vi "ADC_main.vi"() -> ()   [LabVIEW 2013]
uses:
  <vilib>/Platform/TimedLoop/XDataNode/timing_clust.ctl
  <vilib>/Platform/TimedLoop/XDataNode/nitl_modes.ctl
  <vilib>/Platform/TimedLoop/XDataNode/wakeup.ctl
  <vilib>/rvi/Emulation/niFpgaSctlEmulationGetInTimedLoop.vi
  <vilib>/rvi/Emulation/niFpgaEmulationReportErrorSimple.vi
  <vilib>/rvi/Emulation/niFpgaGetClockAttributes.vi
  <vilib>/rvi/Emulation/niFpgaCriticalErrorInLSC.vi
  <vilib>/rvi/FIFO/Fifo_Resource/nirvififoEmulationWriteFpgaImpl.vi
  <vilib>/rvi/DataTransferAndStorage/Container/Common/niFpgaContainerGetUniqueNameForEmu.vi
  <vilib>/rvi/FIFO/Fifo_Resource/nirvififoEmulationReadFpgaImpl.vi
  <vilib>/rvi/Emulation/niFpgaProcessEmulError.vi
  <vilib>/rvi/FIFO/Fifo_Resource/nirvififoEmulationClearFpgaImpl.vi
  <vilib>/rvi/FIFO/Fifo_Resource/nirvififoEmulationGetNumberOfElementsToReadFpgaImpl.vi
  <vilib>/Platform/TimedLoop/XDataNode/XDataNode.xnode
  <vilib>/rvi/DataTransferAndStorage/Container/XNode/niFpgaContainer.xnode
  <vilib>/rvi/FIFO/Fifo_Resource/nirvififoEmulationWrite.vi
  <vilib>/rvi/FIFO/Fifo_Resource/nirvififoEmulationRead.vi
  <vilib>/rvi/FIFO/Fifo_Resource/nirvififoEmulationClear.vi
  <vilib>/rvi/FIFO/Fifo_Resource/nirvififoEmulationGetNumberOfElementsToRead.vi
  <vilib>/Platform/TimedLoop/XDataNode/XDNodeRunTimeDep.lvlib
panel:
  out "Timed out":bool
  out "Config":u16[](array[numeric])
  out "temp FIFO":u32
  out "config FIFO":u32
  out "output":bool
  out "ticks":i32
  out "acqu loops 2":i16
  out "avg loop":i16
  out "acqu loops":i16
  out "Number of Elements to Read":u32
  out "Data [i]":fxp<+/-,26,5>
  in  "trigger resets":i32
  in  "clock resets":i32
  in  "manual trigger":bool
  in  "acquisition":bool
  in  "get order":bool
  in  "order in":u64=434597364041252864
  in  "mode":enum16{"ramp", "RT"}(ring)=enum."RT"
  in  "avg on":bool
  out "err 2":errorcluster
  in  "Nchannels":u32=2
  out "err 1":errorcluster
  in  "avg per pt":u32=10
  out "trigged":bool
  in  "edge":enum8{"falling", "rising", "both"}(ring)=enum."both"
  in  "Trigger":i16
  in  "samples to read":u32=6
  in  "stop":bool=TRUE
  in  "clock divider":u32=160
  out "clock tick":bool
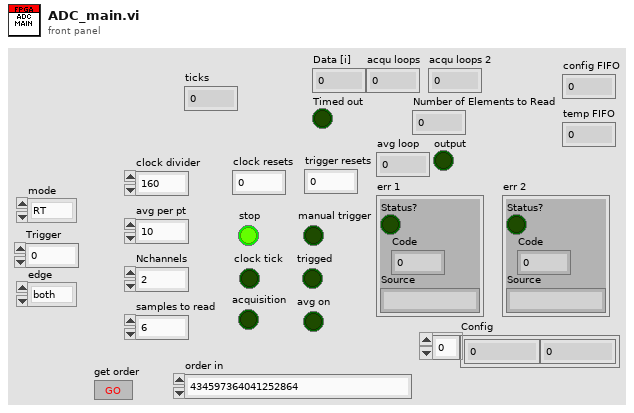
[diagram p1: front panel]
types:
  T1 = typedef "XDNodeRunTimeDep.lvlib/timing_clust.ctl" = cluster{"Expected End [f-1]":u64, "Actual End [f-1]":u64, "Finished Late? [f-1]":bool, "Expected End [i-1]":u64, "Actual End [i-1]":u64, "Finished Late? [i-1]":bool, "Expected Start [i]":u64, "Actual Start [i]":u64, "Expected Start [f]":u64, "Actual Start [f]":u64, "Source Name":string, "Structure Name":string, "Period":i64, "Deadline":i64, "Offset":i64, "Start":i64, "Priority":i32, "Timeout":i32, "Mode":T2, "Wakeup Reason":T3, "Error":errorcluster, "Source Type":string, "Secondary Source Type":string, "Global End Time":u64, "Global Start Time":u64, "Frame Duration":u64, "Iteration Duration":u64, "Assigned CPU":i32, "I/O Scan Engine Mode":u32}
  T2 = typedef "XDNodeRunTimeDep.lvlib/nitl_modes.ctl" = enum32{"No Change", "Process missed periods, maintain original phase", "Discard missed periods, maintain original phase", "Process missed periods, ignore original phase", "Discard missed periods, ignore original phase"}
  T3 = typedef "XDNodeRunTimeDep.lvlib/wakeup.ctl" = enum32{"Normal", "Aborted", "Asynchronous wakeup", "Timing source error", "Timed loop error", "Timeout"}
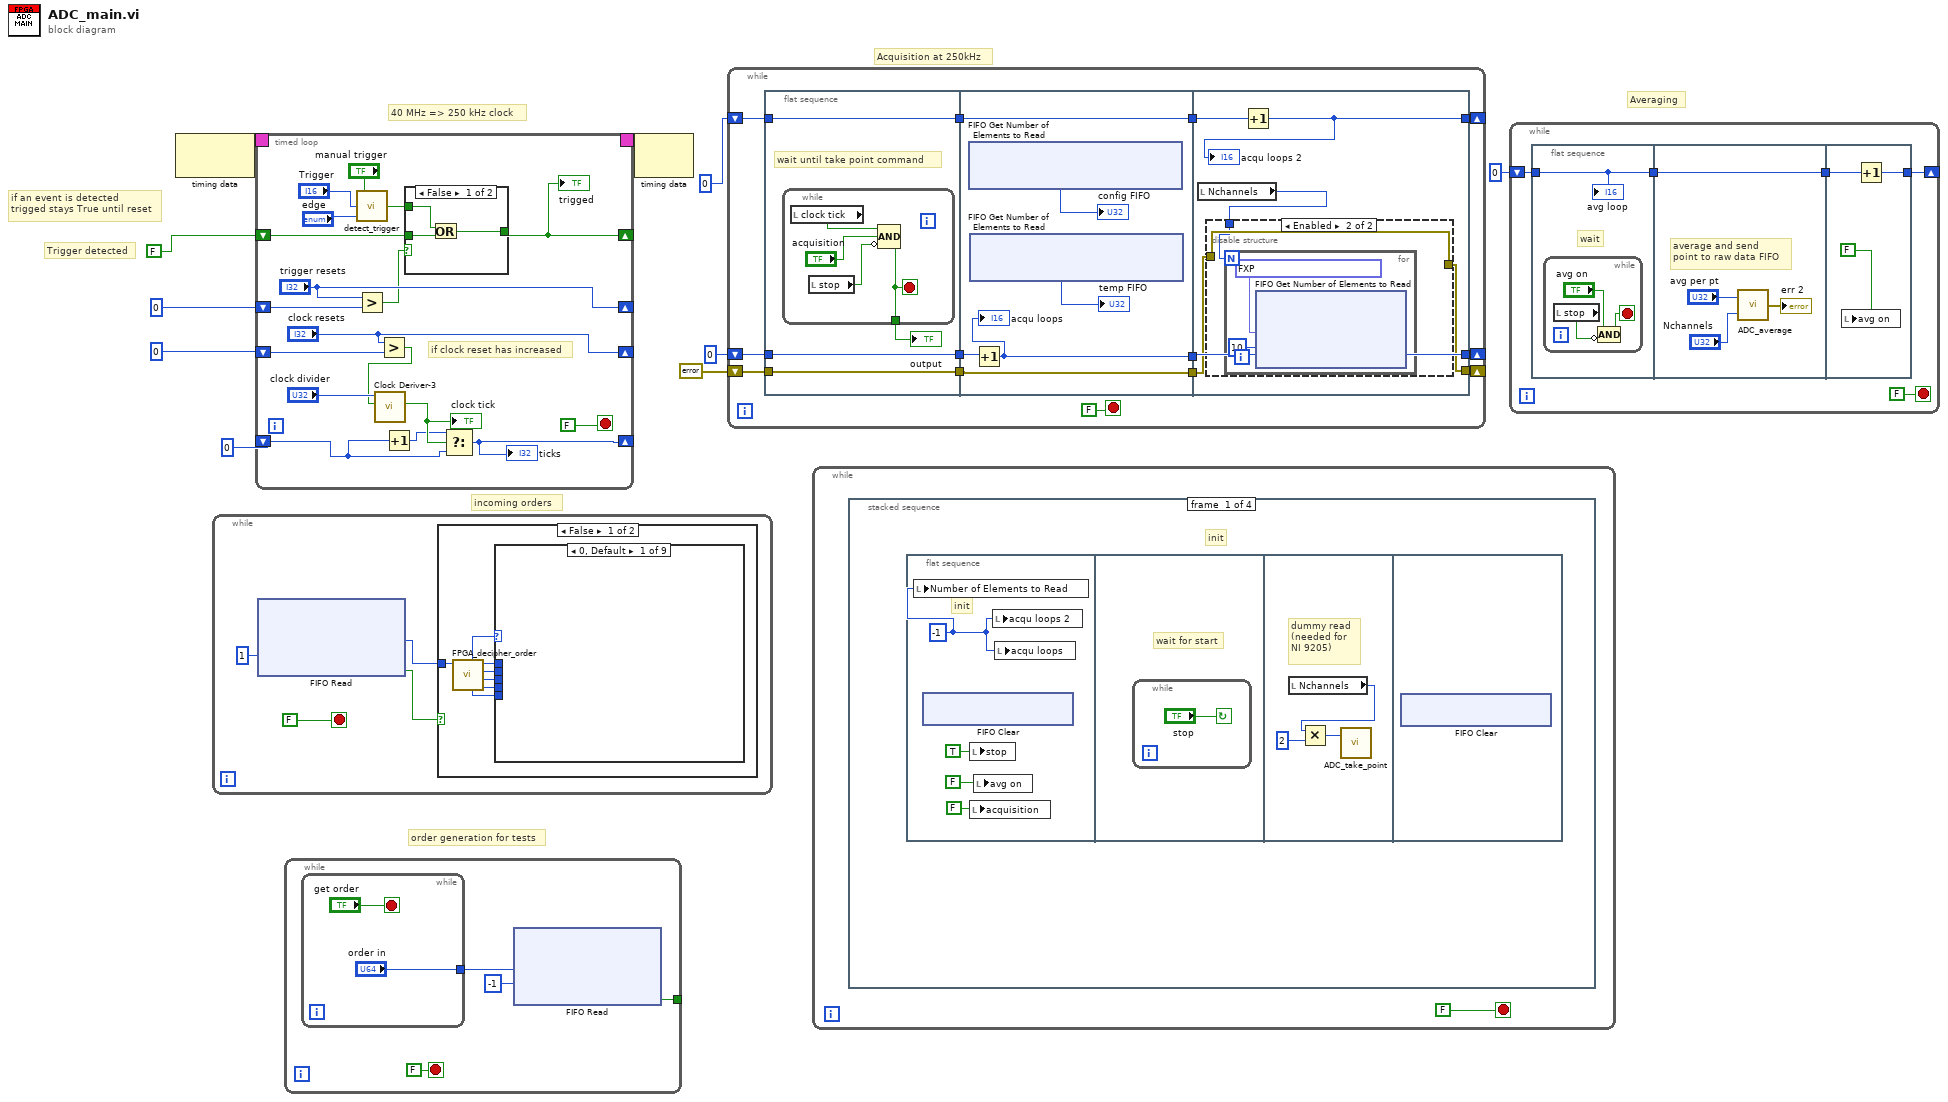
[diagram p0: block diagram]
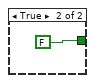
[diagram p2: hidden frame]
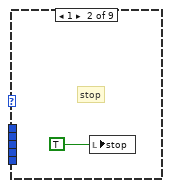
[diagram p3: hidden frame]
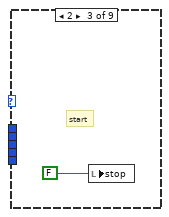
[diagram p4: hidden frame]
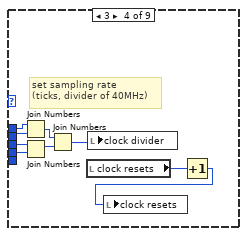
[diagram p5: hidden frame]
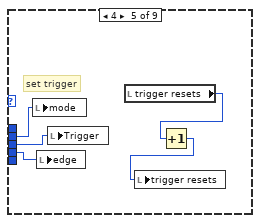
[diagram p6: hidden frame]
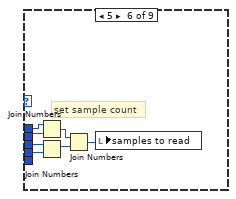
[diagram p7: hidden frame]
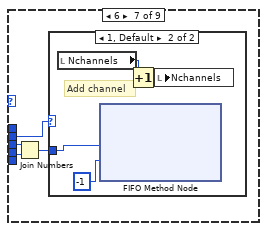
[diagram p8: hidden frame]
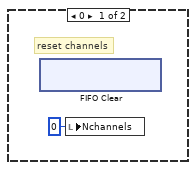
[diagram p9: hidden frame]
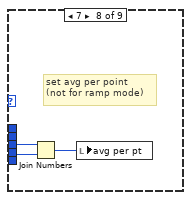
[diagram p10: hidden frame]
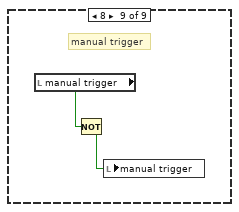
[diagram p11: hidden frame]
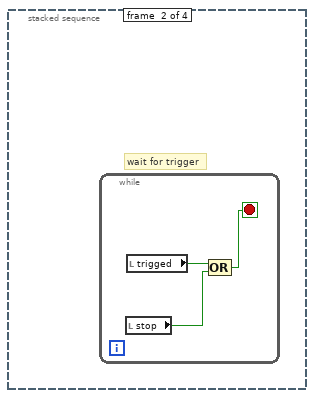
[diagram p13: hidden frame]
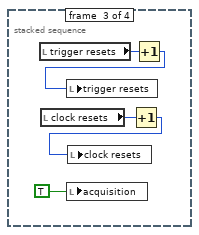
[diagram p14: hidden frame]
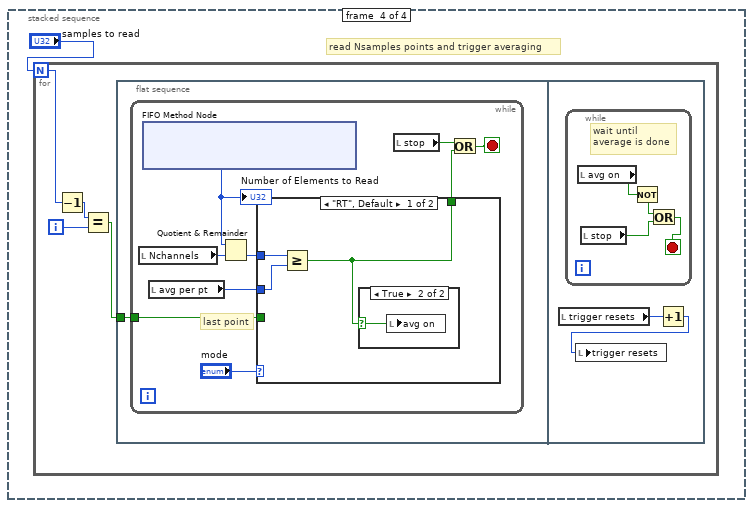
[diagram p15: hidden frame]
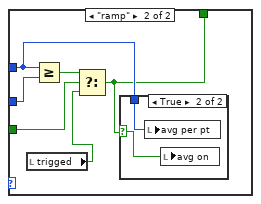
[diagram p17: hidden frame]
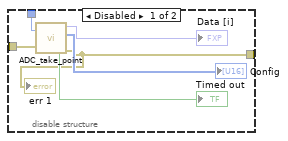
[diagram p19: hidden frame]
diagram:
  # "if an event is detected\ntrigged stays True until reset"
  # "Trigger detected"
  # "40 MHz => 250 kHz clock"
  # "incoming orders"
  # "order generation for tests"
  # "Averaging"
  # "Acquisition at 250kHz"
  n1 = node-c288() -> (w10:T1)  [unwired: 1 in]
  n2 = while {
    stop <- FALSE stop-if-true
    n3 = xnode ("FIFO Read")("Timeout"=1) -> ("Element"=w13:u64, "Timed Out?"=w11:bool)  [unwired: 1 in, 1 out]
    n4 = case shown="False" w11 {
      tunnel: w13 -> [w15 _]
      frame False {
        n5 = call "FPGA_decipher_order.vi"("order in"=w15) -> ("data 1"=w20:u8, "data 2"=w19:u8, "data 3"=w17:u8, "data 4"=w18:u8, "RFU 2"=w16:u8, "order out"=w21:u8)  [unwired: 5 out]
        n6 = case shown="0, Default" w21 {
          tunnel: w20 -> [_ _ _ w31 w37 w43 w47 w55 _]
          tunnel: w19 -> [_ _ _ w32 w35 w44 w48 w56 _]
          tunnel: w18 -> [_ _ _ w30 _ w42 _ _ _]
          tunnel: w17 -> [_ _ _ w29 w36 w41 w45 _ _]
          tunnel: w16 -> [_ _ _ _ _ _ _ _ _]
          frame 0, Default {
          }
          frame 1 {
            # "stop"
            n7 = local write "stop"(TRUE ("Stop seq")) -> ()
          }
          frame 2 {
            # "start"
            n8 = local write "stop"(FALSE ("Stop seq")) -> ()
          }
          frame 3 {
            # "set sampling rate \n(ticks, divider of 40MHz)"
            n9 = Join Numbers(hi=w30, lo=w29) -> ((hi.lo)=w28:u16)
            n10 = Join Numbers(hi=w32, lo=w31) -> ((hi.lo)=w27:u16)
            n11 = Join Numbers(hi=w28, lo=w27) -> ((hi.lo)=w26:u32)
            n12 = local read "clock resets"() -> (w25:i32)
            n13 = local write "clock divider"(w26) -> ()
            n14 = Increment(x=w25) -> (x+1=w24:i32)
            n15 = local write "clock resets"(w24) -> ()
          }
          frame 4 {
            # "set trigger"
            n16 = local write "mode"(w36) -> ()
            n17 = local write "edge"(w37) -> ()
            n18 = local write "Trigger"(w35) -> ()
            n19 = local read "trigger resets"() -> (w34:i32)
            n20 = Increment(x=w34) -> (x+1=w33:i32)
            n21 = local write "trigger resets"(w33) -> ()
          }
          frame 5 {
            # "set sample count"
            n22 = Join Numbers(hi=w42, lo=w41) -> ((hi.lo)=w40:u16)
            n23 = Join Numbers(hi=w44, lo=w43) -> ((hi.lo)=w39:u16)
            n24 = Join Numbers(hi=w40, lo=w39) -> ((hi.lo)=w38:u32)
            n25 = local write "samples to read"(w38) -> ()
          }
          frame 6 {
            n26 = Join Numbers(hi=w48, lo=w47) -> ((hi.lo)=w46:u16)
            n27 = case shown="1, Default" w45 {
              tunnel: w46 -> [_ w52]
              frame 0 {
                # "reset channels"
                n28 = xnode ("FIFO Clear")() -> ()  [unwired: 1 in, 1 out]
                n29 = local write "Nchannels"(0 ("Nchannels")) -> ()
              }
              frame 1, Default {
                # "Add channel"
                n30 = local read "Nchannels"() -> (w50:u32)
                n31 = xnode ("FIFO Method Node")("Element"=w52, "Timeout"=-1) -> ()  [unwired: 2 in, 3 out]
                n32 = Increment(x=w50) -> (x+1=w51:u32)
                n33 = local write "Nchannels"(w51) -> ()
              }
            }
          }
          frame 7 {
            # "set avg per point\n(not for ramp mode)"
            n34 = Join Numbers(hi=w56, lo=w55) -> ((hi.lo)=w54:u16)
            n35 = local write "avg per pt"(w54) -> ()
          }
          frame 8 {
            # "manual trigger"
            n36 = local read "manual trigger"() -> (w58:bool)
            n37 = Not(x=w58) -> (.not. x?=w57:bool)
            n38 = local write "manual trigger"(w57) -> ()
          }
        }
      }
      frame True {
      }
    }
  }
  n39 = timed-loop {
    timing: w10 -> [_]
    timing-out: [_] -> w9
    shift-right: [w74] -> _
    shift-left: FALSE ("reset trigger") -> [w75]
    shift-right: ["clock resets"] -> _
    shift-left: 0 ("clock resets") -> [w68]
    shift-right: ["trigger resets"] -> _
    shift-left: 0 ("trigger resets") -> [w65]
    shift-right: [w59] -> _
    shift-left: 0 -> [w60]
    stop <- FALSE stop-if-true
    # "if clock reset has increased"
    n40 = call "detect_trigger.vi"("edge"="edge", "trigger"="Trigger", "manual trigger"="manual trigger") -> ("trigged"=w73:bool)
    n41 = Greater?(x="trigger resets", y=w65) -> (0:w63:bool)
    n42 = Greater?(x="clock resets", y=w68) -> (0:w67:bool)
    n43 = call "Clock Deriver-3.vi"("reset"=w67, "Divisor"="clock divider") -> ("Clock Out"=w62:bool)  [unwired: 9 in]
    "clock tick" <- w62
    n44 = Increment(x=w60) -> (x+1=w61:i32)
    n45 = case shown="False" w63 {
      tunnel: w73 -> [w79 _]
      tunnel: w75 -> [w78 _]
      tunnel: [w77 FALSE] -> w74
      frame False {
        n46 = Or(x=w79, y=w78) -> (x .or. y?=w77:bool)
      }
      frame True {
      }
    }
    "trigged" <- w74
    n47 = Select(t=w61, s=w62, f=w60) -> (s? t:f=w59:i32)
    "ticks" <- w59
  }
  n48 = while {
    tunnel: [w83] -> _
    stop <- FALSE stop-if-true
    n49 = while {
      tunnel: ["order in"] -> w84
      stop <- "get order" stop-if-true
    }
    n50 = xnode ("FIFO Read")("Element"=w84, "Timeout"=-1) -> ("Timed Out?"=w83:bool)  [unwired: 1 in, 1 out]
  }
  n51 = node-c288(w9) -> ()  [unwired: 1 out]
  n52 = while {
    shift-right: [w99] -> _
    shift-left: i16 0 -> [w100]
    shift-right: [w93] -> _
    shift-left: i16 0 -> [w98]
    shift-right: [w92] -> _
    shift-left: errorcluster {"Status?"=FALSE, "Code"=0, "Source"=""} ("err out") -> [w90]
    stop <- FALSE stop-if-true
    n53 = flat-sequence {
      tunnel: [w105] -> w97
      tunnel: w100 -> [w105]
      tunnel: w98 -> [w103]
      tunnel: [w103] -> w95
      tunnel: w90 -> [w102]
      tunnel: [w102] -> w89
      tunnel: w97 -> [w115]
      tunnel: [w115] -> w96
      tunnel: w95 -> [w114]
      tunnel: [w113] -> w94
      tunnel: [w110] -> w91
      tunnel: w89 -> [w110]
      tunnel: w96 -> [w120]
      tunnel: [w119] -> w99
      tunnel: w94 -> [w118]
      tunnel: [w118] -> w93
      tunnel: [w116] -> w92
      tunnel: w91 -> [w117]
      frame #0 {
        # "wait until take point command"
        n54 = while {
          tunnel: [w106] -> w104
          stop <- w106 stop-if-true
          n55 = local read "clock tick"() -> (w109:bool)
          n56 = local read "stop"() -> (w107:bool)
          n57 = Compound Arithmetic op=AND(w109, "acquisition", invert w107) -> (w106:bool)
        }
        "output" <- w104
      }
      frame #1 {
        n58 = xnode ("FIFO Get Number of Elements to Read")() -> ("Number of Elements to Read"=→"config FIFO":u32)  [unwired: 1 in, 1 out]
        n59 = xnode ("FIFO Get Number of Elements to Read")() -> ("Number of Elements to Read"=→"temp FIFO":u32)  [unwired: 1 in, 1 out]
        n60 = Increment(x=w114) -> (x+1=w113:i16)
        "acqu loops" <- w113
      }
      frame #2 {
        n61 = local read "Nchannels"() -> (w121:u32)
        n62 = disable-structure shown="Enabled" {
          disable-tunnel: w121 -> [w127 w128]
          disable-tunnel: w117 -> [w123 w129]
          disable-tunnel: [w122 w129] -> w116
          frame Disabled {
            n63 = call "ADC_take_point.vi"("Nchannels"=w127, "error in"=w123) -> ("Data [i]"=→"Data [i]":fxp<+/-,26,5>, "Config"=→"Config":u16[], "Timed out"=→"Timed out":bool, "err out"=w122:errorcluster)
            "err 1" <- w122
          }
          frame Enabled {
            n64 = for {
              N: w128 -> [_]
              n65 = xnode ("FIFO Get Number of Elements to Read")("Element"=fxp<+/-,26,5> -0.09999990463256836 ("fixed-point"), "Timeout"=10) -> ()  [unwired: 1 in, 2 out]
            }
          }
        }
        n66 = Increment(x=w120) -> (x+1=w119:i16)
        "acqu loops 2" <- w119
      }
    }
  }
  n67 = while {
    stop <- FALSE stop-if-true
    n68 = stacked-sequence {
      frame #0 {
        # "init"
        n69 = flat-sequence {
          frame #0 {
            w133 = i16 -1 ("acqu loops")
            # "init"
            n70 = local write "Number of Elements to Read"(w133) -> ()
            n71 = xnode ("FIFO Clear")() -> ()  [unwired: 1 in, 1 out]
            n72 = local write "stop"(TRUE ("stop")) -> ()
            n73 = local write "acquisition"(FALSE) -> ()
            n74 = local write "avg on"(FALSE) -> ()
            n75 = local write "acqu loops 2"(w133) -> ()
            n76 = local write "acqu loops"(w133) -> ()
          }
          frame #1 {
            # "wait for start"
            n77 = while {
              stop <- "stop" continue-if-true
            }
          }
          frame #2 {
            # "dummy read\n(needed for\nNI 9205)"
            n78 = local read "Nchannels"() -> (w140:u32)
            n79 = Multiply(x=w140, y=u32 2) -> (x*y=w138:u32)
            n80 = call "ADC_take_point.vi"("Nchannels"=w138) -> ()  [unwired: 1 in, 4 out]
          }
          frame #3 {
            n81 = xnode ("FIFO Clear")() -> ()  [unwired: 1 in, 1 out]
          }
        }
      }
      frame #1 {
        # "wait for trigger"
        n82 = while {
          stop <- w142 stop-if-true
          n83 = local read "stop"() -> (w143:bool)
          n84 = local read "trigged"() -> (w141:bool)
          n85 = Compound Arithmetic op=OR(w141, w143) -> (w142:bool)
        }
      }
      frame #2 {
        n86 = local read "trigger resets"() -> (w147:i32)
        n87 = local read "clock resets"() -> (w145:i32)
        n88 = local write "acquisition"(TRUE ("acquisition")) -> ()
        n89 = Increment(x=w145) -> (x+1=w144:i32)
        n90 = local write "clock resets"(w144) -> ()
        n91 = Increment(x=w147) -> (x+1=w146:i32)
        n92 = local write "trigger resets"(w146) -> ()
      }
      frame #3 {
        # "read Nsamples points and trigger averaging"
        n93 = for {
          N: "samples to read" -> [w150]
          i -> [w153]
          n94 = Decrement(x=w150) -> (x-1=w152:i32)
          n95 = Equal?(x=w152, y=w153) -> (x = y?=w151:bool)
          n96 = flat-sequence {
            tunnel: w151 -> [w154]
            frame #0 {
              n97 = while {
                tunnel: w154 -> [w158]
                stop <- w155 stop-if-true
                # "last point"
                n98 = local read "Nchannels"() -> (w160:u32)
                n99 = xnode ("FIFO Method Node")() -> ("Number of Elements to Read"=w159:u32)  [unwired: 1 in, 1 out]
                "Number of Elements to Read" <- w159
                n100 = local read "avg per pt"() -> (w163:u32)
                n101 = Quotient & Remainder(x=w159, y=w160) -> (floor(x/y)=w162:u32)  [unwired: 1 out]
                n102 = case shown="\"RT\", Default" "mode" {
                  tunnel: w162 -> [w166 w169]
                  tunnel: w163 -> [w165 w173]
                  tunnel: [w164 w168] -> w156
                  tunnel: w158 -> [_ w171]
                  frame "RT", Default {
                    n103 = Greater Or Equal?(x=w166, y=w165) -> (x >= y?=w164:bool)
                    n104 = case shown="True" w164 {
                      selector: w164 -> [_ w167]
                      frame False {
                      }
                      frame True {
                        n105 = local write "avg on"(w167) -> ()
                      }
                    }
                  }
                  frame "ramp" {
                    n106 = local read "trigged"() -> (w170:bool)
                    n107 = Greater Or Equal?(x=w169, y=w173) -> (x >= y?=w172:bool)
                    n108 = Select(t=w172, s=w171, f=w170) -> (s? t:f=w168:bool)
                    n109 = case shown="True" w168 {
                      selector: w168 -> [_ w174]
                      tunnel: w169 -> [_ w175]
                      frame False {
                      }
                      frame True {
                        n110 = local write "avg per pt"(w175) -> ()
                        n111 = local write "avg on"(w174) -> ()
                      }
                    }
                  }
                }
                n112 = local read "stop"() -> (w157:bool)
                n113 = Or(x=w157, y=w156) -> (x .or. y?=w155:bool)
              }
            }
            frame #1 {
              n114 = local read "trigger resets"() -> (w176:i32)
              n115 = while {
                stop <- w178 stop-if-true
                # "wait until \naverage is done"
                n116 = local read "avg on"() -> (w179:bool)
                n117 = local read "stop"() -> (w181:bool)
                n118 = Not(x=w179) -> (.not. x?=w180:bool)
                n119 = Or(x=w180, y=w181) -> (x .or. y?=w178:bool)
              }
              n120 = Increment(x=w176) -> (x+1=w177:i32)
              n121 = local write "trigger resets"(w177) -> ()
            }
          }
        }
      }
    }
  }
  n122 = while {
    shift-right: [w182] -> _
    shift-left: i16 0 -> [w185]
    stop <- FALSE stop-if-true
    n123 = flat-sequence {
      tunnel: w185 -> [w187]
      tunnel: [w187] -> w183
      tunnel: [w191] -> w184
      tunnel: w183 -> [w191]
      tunnel: w184 -> [w196]
      tunnel: [w195] -> w182
      frame #0 {
        # "wait"
        n124 = while {
          stop <- w188 stop-if-true
          n125 = local read "stop"() -> (w189:bool)
          n126 = Compound Arithmetic op=AND("avg on", invert w189) -> (w188:bool)
        }
        "avg loop" <- w187
      }
      frame #1 {
        # "average and send \npoint to raw data FIFO"
        n127 = call "ADC_average.vi"("Nchannels"="Nchannels", "avg per pt"="avg per pt") -> ("err out"=→"err 2":errorcluster)
      }
      frame #2 {
        n128 = local write "avg on"(FALSE) -> ()
        n129 = Increment(x=w196) -> (x+1=w195:i16)
      }
    }
  }
